vi "ABR3-Plot Waveforms.vi"(0 "Array":dbl[][](array[numeric]), 1 "ControlVal":dbl=nan, 2 "graph ref":refnum<vi>, 5 "dt (us)":dbl, 7 "Normalize traces":bool, 9 "Seqvals":dbl[](array[numeric]), 11 "error in (no error)":errorcluster, 12 "InnerVals":dbl[](array[numeric]), 13 "Threshold":dbl=nan) -> (15 "error out":errorcluster)   [LabVIEW 2020]
uses:
  epl-vi-lib/Utility VIs/Math VIs/LinSpace (x0-dx-npts).vi
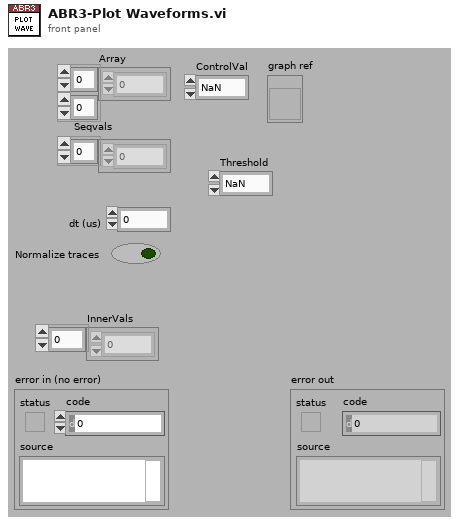
[diagram p1: front panel]
types:
  T1 = cluster{"Name":string, "Color":u32, "Style":u8, "Point Style":u8, "Name Visible":bool, "Allow Drag":bool, "Annotation Mode":u32, "Plot":i32, "Index":i32, "Position":cluster{"X":dbl, "Y":dbl}, "X Scale":u32, "Y Scale":u32, "Show Arrow":bool, "Lock Name":bool, "Plot Area":i32, "Label Offset":cluster{"X":dbl, "Y":dbl}}
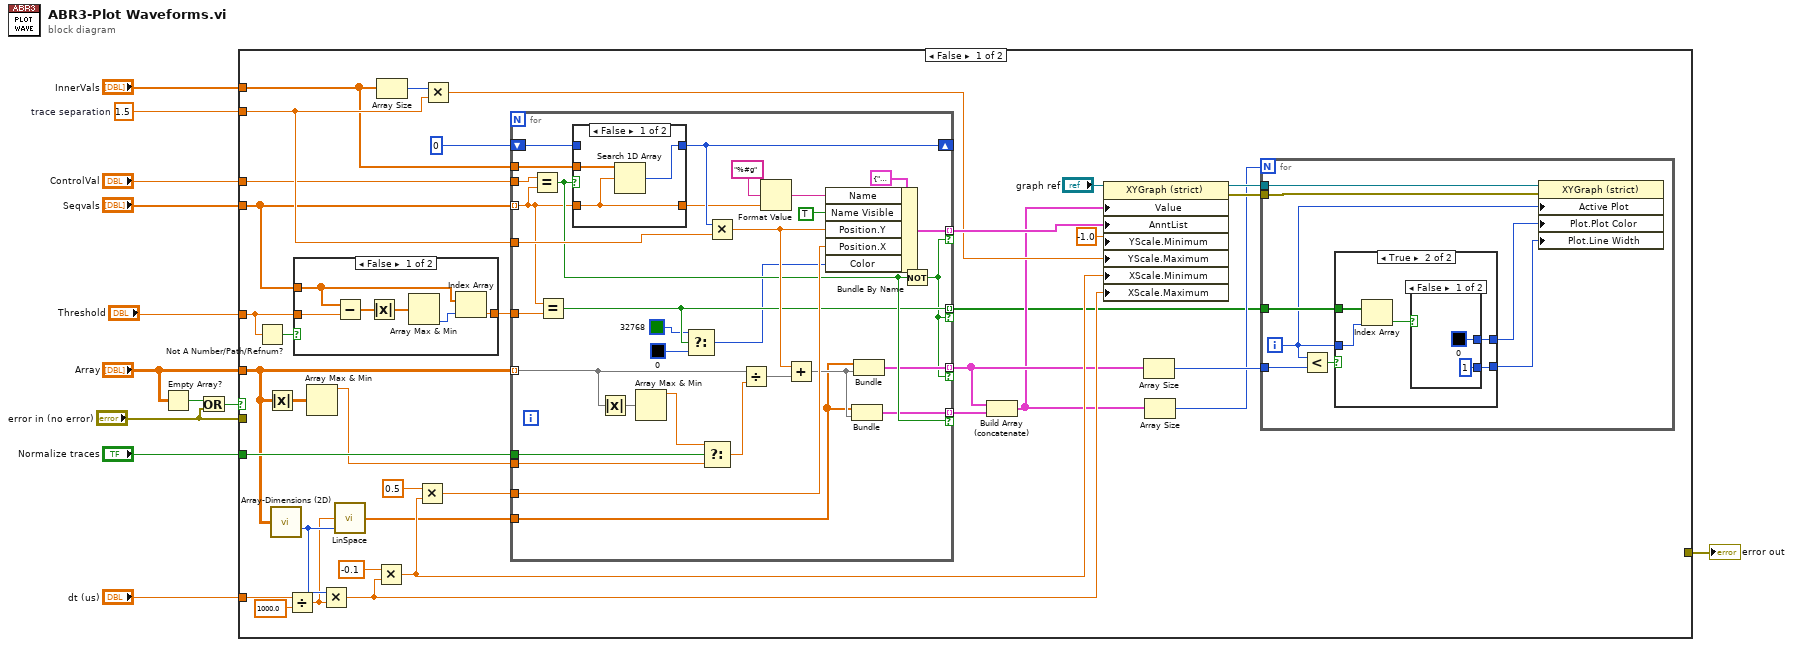
[diagram p0: block diagram]
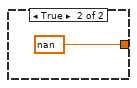
[diagram p2: hidden frame]
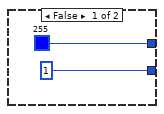
[diagram p3: hidden frame]
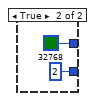
[diagram p4: hidden frame]
diagram:
  w9 = 1.5  # trace separation
  n1 = Empty Array?(array="Array") -> (empty?=w6:bool)
  n2 = Or(x=w6, y="error in (no error)") -> (x .or. y?=w4:bool)
  n3 = case shown="False" w4 {
    tunnel: "Array" -> [w37 _]
    tunnel: "dt (us)" -> [w47 _]
    tunnel: [_ w111] -> w11
    tunnel: "Seqvals" -> [w19 _]
    tunnel: w9 -> [w42 _]
    tunnel: "Normalize traces" -> [w40 _]
    tunnel: "InnerVals" -> [w31 _]
    tunnel: "error in (no error)" -> [_ w111]
    tunnel: "ControlVal" -> [w30 _]
    tunnel: "Threshold" -> [w14 _]
    frame False {
      n4 = Not A Number/Path/Refnum?(number/path/refnum=w14) -> (NaN/Path/Refnum?=w13:bool)
      n5 = Absolute Value(x=w37) -> (abs(x)=w39:dbl[][])
      n6 = call "Array-Dimensions (2D).vi"("2D Array"=w37) -> ("# columns"=w27:i32)  [unwired: 13 in, 1 out]
      n7 = Divide(x=w47, y=1000.0) -> (x/y=w25:dbl)
      n8 = case shown="False" w13 {
        tunnel: w19 -> [w50 _]
        tunnel: [w48 nan] -> w18
        tunnel: w14 -> [w51 _]
        frame False {
          n9 = Subtract(x=w50, y=w51) -> (x-y=w53:dbl[])
          n10 = Absolute Value(x=w53) -> (abs(x)=w52:dbl[])
          n11 = Array Max & Min(array=w52) -> (min index (indices)=w49:i32)  [unwired: 3 out]
          n12 = Index Array(array=w50, index=w49) -> (element=w48:dbl)
        }
        frame True {
        }
      }
      n13 = Array Max & Min(array=w39) -> (max value=w38:dbl)  [unwired: 3 out]
      n14 = Multiply(x=w27, y=w25) -> (x*y=w36:dbl)
      n15 = call-poly "LinSpace.vi"("npts"=w27, "dx"=w25) -> ("Array"=w26:dbl[])  [unwired: 2 in, 1 out]
      n16 = Multiply(x=-0.1, y=w36) -> (x*y=w33:dbl)
      n17 = Array Size(array=w31) -> (size(s)=w32:i32)
      n18 = Multiply(x=0.5, y=w33) -> (x*y=w29:dbl)
      n19 = Multiply(x=w32, y=w42) -> (x*y=w41:dbl)
      n20 = for {
        tunnel: w37 -> [w104] mode=indexing
        tunnel: [w83] -> w23 mode=indexing if=w74
        tunnel: w19 -> [w79] mode=indexing
        tunnel: [w100] -> w44 mode=indexing if=w74
        tunnel: w42 -> [w99]
        tunnel: w40 -> [w96]
        tunnel: w38 -> [w93]
        tunnel: w31 -> [w91]
        tunnel: w30 -> [w90]
        tunnel: w29 -> [w89]
        shift-right: [w88] -> _
        shift-left: 0 -> [w87]
        tunnel: [w82] -> w24 mode=indexing if=w84
        tunnel: w26 -> [w81]
        tunnel: w18 -> [w80]
        tunnel: [w78] -> w15 mode=indexing if=w74
        n21 = Equal?(x=w90, y=w79) -> (x = y?=w84:bool)
        n22 = Equal?(x=w79, y=w80) -> (x = y?=w78:bool)
        n23 = case shown="False" w84 {
          tunnel: w91 -> [w108 _]
          tunnel: [w107 w110] -> w88
          tunnel: w79 -> [w106 w109]
          tunnel: w87 -> [_ w110]
          tunnel: [w106 w109] -> w86
          frame False {
            n24 = Search 1D Array(1D array=w108, element=w106) -> (index of element=w107:i32)  [unwired: 1 in]
          }
          frame True {
          }
        }
        n25 = Absolute Value(x=w104) -> (abs(x)=w105:dbl[])
        n26 = Array Max & Min(array=w105) -> (max value=w95:dbl)  [unwired: 3 out]
        n27 = Select(t=u32 32768, s=w78, f=u32 0) -> (s? t:f=w75:u32)
        n28 = Select(t=w95, s=w96, f=w93) -> (s? t:f=w94:dbl)
        n29 = Multiply(x=w88, y=w99) -> (x*y=w98:dbl)
        n30 = Divide(x=w104, y=w94) -> (x/y=w97:dbl[])
        n31 = Format Value(format string="%#g", value (0)=w86) -> (output string=w101:string)  [unwired: 1 in]
        n32 = Add(x=w98, y=w97) -> (x+y=w85:dbl[])
        n33 = Bundle By Name(cluster=T1 {"Name"="", "Color"=0, "Style"=0, "Point Style"=0, "Name Visible"=FALSE, "Allow Drag"=FALSE, "Annotation Mode"=0, "Plot"=0, "Index"=0, "Position"={"X"=0.0, "Y"=0.0}, "X Scale"=0, "Y Scale"=0, "Show Arrow"=FALSE, "Lock Name"=FALSE, "Plot Area"=0, "Label Offset"={"X"=0.0, "Y"=0.0}} ("dummy annotation cluster\n(so we can bundle by name)"), "Name"=w101, "Name Visible"=TRUE, "Position.Y"=w98, "Position.X"=w89, "Color"=w75) -> (w100:T1)
        n34 = Bundle("Array"=w81, w85) -> (w82:cluster{"Array":dbl[], dbl[]})  [unwired: 1 in]
        n35 = Bundle("Array"=w81, w85) -> (w83:cluster{"Array":dbl[], dbl[]})  [unwired: 1 in]
        n36 = Not(x=w84) -> (.not. x?=w74:bool)
      }
      n37 = Build Array (concatenate)(w23, w24) -> (w17:cluster{"Array":dbl[], dbl[]}[])
      n38 = property class="XYGraph (strict)"(reference="graph ref", "Value"=w17, "AnntList"=w44, "YScale.Minimum"=-1.0 ("Y Scale.Range:Minimum"), "YScale.Maximum"=w41, "XScale.Minimum"=w33, "XScale.Maximum"=w36) -> (reference out=w22:refnum<vi>, error out=w21:errorcluster)  [unwired: 1 in]
      n39 = Array Size(array=w23) -> (size(s)=w20:i32)
      n40 = Array Size(array=w17) -> (size(s)=w16:i32)
      n41 = for {
        N: w16 -> [_]
        tunnel: w22 -> [w62]
        tunnel: w21 -> [w61]
        tunnel: w20 -> [w60]
        tunnel: w15 -> [w57]
        i -> [w56]
        n42 = Less?(x=w56, y=w60) -> (x < y?=w55:bool)
        n43 = case shown="True" w55 {
          tunnel: [u32 255 w69] -> w59
          tunnel: [1 w68] -> w58
          tunnel: w57 -> [_ w67]
          tunnel: w56 -> [_ w65]
          frame False {
          }
          frame True {
            n44 = Index Array(array=w67, index=w65) -> (element=w66:bool)
            n45 = case shown="False" w66 {
              tunnel: [u32 0 u32 32768] -> w69
              tunnel: [1 2] -> w68
              frame False {
              }
              frame True {
              }
            }
          }
        }
        n46 = property class="XYGraph (strict)"(reference=w62, error in=w61, "Active Plot"=w56, "Plot.Plot Color"=w59, "Plot.Line Width"=w58) -> ()  [unwired: 2 out]
      }
    }
    frame True {
    }
  }
  "error out" <- w11
